vi "AutoArmReadyWait.vi"(8 "error in (no error)":errorcluster, 10 "ArmSetpoints":T1, 11 "TimeOut (s)":dbl=99.0) -> (0 "error out":errorcluster)   [LabVIEW 2023]
doc: "Wrapper class for auto do nothing and wait\nInput:\n -- error in -- Cluster \n -- time out -- Double -- how long to wait B4 quitting\nOutput:\n -- error out -- Cluster"
uses:
  <vilib>/Rock Robotics/WPI/ThirdParty/JAS_Junk/TrajLib/Trajectory_Library.lvlib
  Shoulder/ShoulderGetSetpointEnum.ctl
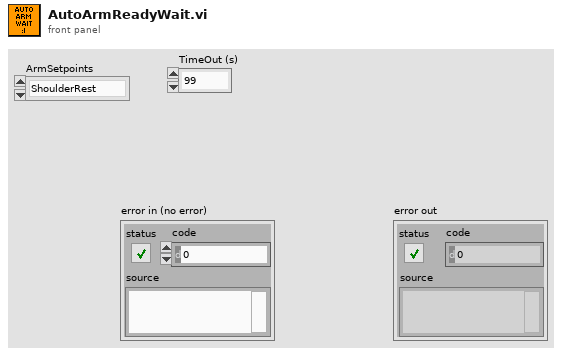
[diagram p1: front panel]
types:
  T1 = typedef "ShoulderGetSetpointEnum.ctl" = enum16{"ShoulderRest", "ShoulderSpeaker", "ShoulderAmp"}
  T2 = typedef "Trajectory_Library.lvlib/TIMER.ctl" = cluster{"StartTime":dbl, "Accumulated TIme":dbl, "Running":bool, "semaphore":T3}
  T3 = typedef "Semaphore RefNum" = refnum<k1>
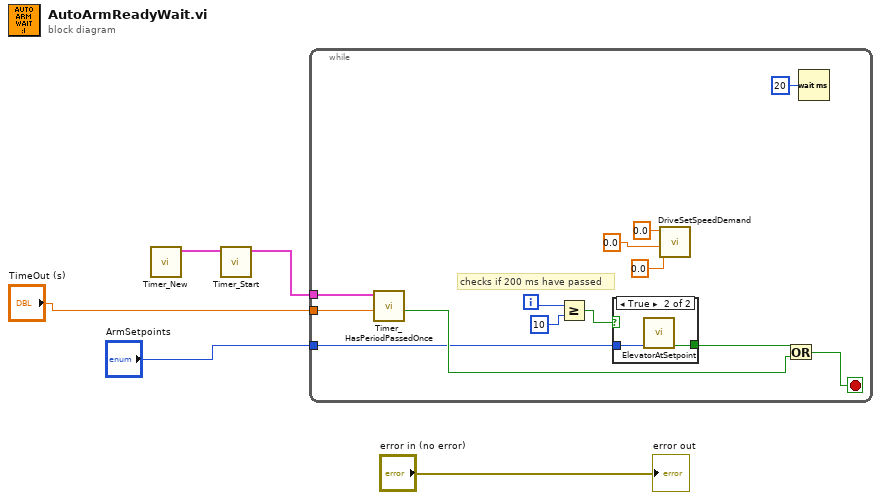
[diagram p0: block diagram]
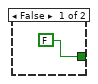
[diagram p2: hidden frame]
diagram:
  n1 = call <vilib>:"Timer_New.vi"() -> ("TIMER"=w4:T2)  [unwired: 11 in]
  n2 = call <vilib>:"Timer_Start.vi"("in Timer"=w4) -> ("out Timer"=w3:T2)  [unwired: 10 in]
  n3 = while {
    tunnel: w3 -> [w18]
    tunnel: "TimeOut (s)" -> [w17]
    tunnel: "ArmSetpoints" -> [w6]
    i -> [w9]
    stop <- w10 stop-if-true
    # "checks if 200 ms have passed"
    n4 = call <vilib>:"Timer_HasPeriodPassedOnce.vi"("Period"=w17, "in Timer"=w18) -> ("Expired"=w11:bool)  [unwired: 7 in, 2 out]
    n5 = Greater Or Equal?(x=w9, y=10) -> (x >= y?=w8:bool)
    n6 = case shown="True" w8 {
      tunnel: [FALSE w21] -> w12
      tunnel: w6 -> [_ w20]
      frame False {
      }
      frame True {
        n7 = call "ElevatorAtSetpoint.vi"("SholdrSetpoints"=w20) -> ("AtSetpoint"=w21:bool)  [unwired: 10 in]
      }
    }
    n8 = call "DriveSetSpeedDemand.vi"("ASpeedDemand (d/s)"=0.0 ("RSpeedDemand (ft/s)"), "YSpeedDemand (ft/s)"=0.0 ("RSpeedDemand (ft/s)"), "XSpeedDemand (ft/s)"=0.0 ("LSpeedDemand (ft/s)")) -> ()  [unwired: 9 in]
    n9 = Or(x=w12, y=w11) -> (x .or. y?=w10:bool)
    n10 = Wait (ms)(milliseconds to wait=u32 20) -> ()  [unwired: 1 out]
  }
  "error out" <- "error in (no error)"
